vi "Parse Persisted Num Array.vi"(11 "file string value":string) -> (2 "valid":bool, 3 "Array of Booleans":dbl[](array[numeric]))   [LabVIEW 2017]
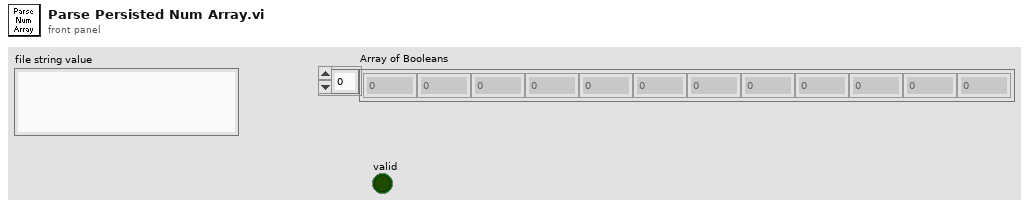
[diagram p1: front panel]
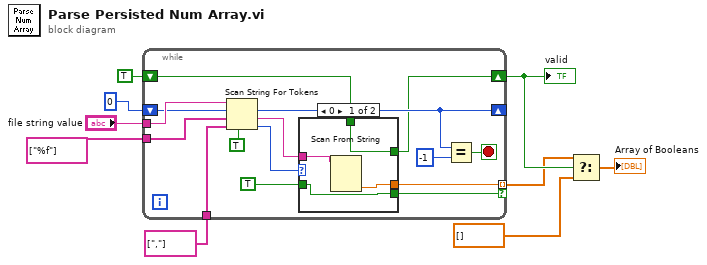
[diagram p0: block diagram]
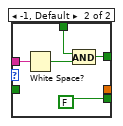
[diagram p2: hidden frame]
diagram:
  n1 = while {
    tunnel: "file string value" -> [w24]
    shift-right: [w19] -> _
    shift-left: 0 -> [w23]
    tunnel: string[] [","] ("delimiters (\\s,\\t,\\r,\\n)") -> [w22]
    tunnel: string[] ["%f"] ("delimiters (\\s,\\t,\\r,\\n)") -> [w21]
    tunnel: [w14] -> w1 mode=indexing if=w13
    shift-right: [w10] -> w4
    shift-left: TRUE ("use cached delim/oper data? (F)") -> [w11]
    stop <- w18 stop-if-true
    n2 = Scan String For Tokens(4:TRUE ("use cached delim/oper data? (F)"), 6:w22, 7:w21, 8:w23, 9:w24) -> (0:w16:i32, 1:w12:string, 2:w19:i32)  [unwired: 1 in, 1 out]
    n3 = case shown="0" w16 {
      tunnel: TRUE -> [w28 _]
      tunnel: [w25 _] -> w14
      tunnel: [w28 FALSE] -> w13
      tunnel: w12 -> [w26 w32]
      tunnel: [w27 w29] -> w10
      tunnel: w11 -> [w27 w30]
      frame 0 {
        n4 = Scan From String(input string=w26) -> (output 1=w25:dbl)  [unwired: 4 in, 3 out]
      }
      frame -1, Default {
        n5 = White Space?(1:w32) -> (0:w31:bool)
        n6 = And(x=w30, y=w31) -> (x .and. y?=w29:bool)
      }
    }
    n7 = Equal?(x=w19, y=-1) -> (x = y?=w18:bool)
  }
  "valid" <- w4
  n8 = Select(t=w1, s=w4, f=dbl[] []) -> (s? t:f=→"Array of Booleans":dbl[])
